vi "PrintTextRead.vi"(0 "No":string, 4 "Time":string, 6 "Date":string, 7 "file path (use dialog)":path=path "E:/NI Program/Merlin try.txt", 8 "Shift":string, 9 "ID":string, 10 "PartNumber":string, 11 "Description":string) -> (1 "FileFound?":bool, 3 "result string":string)   [LabVIEW 2017]
panel:
  in  "PrintMatter":string="\u0010CT~~CD,~CC^~CT~\n^XA~TA080~JSB^LT12^MNW^MTT^PON^PMN^LH0,0^JMA^PR2,2~SD20^JUS^LRN^CI0^XZ\n~DG000.GRF,06400,040,\n,:::::::0FiSFC,0C0iR04,:::::::::::::::::::::::::::::::::::::::::::::::::::::::::::::::::::::::::::::::::::::::::::::::::::::::::::::::::::::::::::::::::::::0FiSFC,:,::::::::::::::^XA\n^MMT\n^PW320\n^LL0152\n^LS0\n^FT0,160^XG000.GRF,1,1^FS\n^FT10,135^A0N,17,16^FH\\^FDDate & Time:^FS\n^FT207,100^A0N,17,16^FH\\^FDID:^FS\n^FT10,98^A0N,17,16^FH\\^FDPart No:^FS\n^FT102,135^A0N,17,16^FH\\^FD01.01.2019 0000^FS\n^FT230,101^A0N,20,19^FH\\^FDoperator^FS\n^FT72,100^A0N,20,19^FH\\^FD123456789^FS\n^FT15,67^A0N,20,19^FH\\^FDFRONT ELECTRIC WR - W501 RH^FS\n^FO4,42^GB297,0,2^FS\n^FT15,31^A0N,17,16^FH\\^FDAditya Auto Products & Engg. (I) Pvt. Ltd.^FS\n^PQ1,0,1,Y^XZ\n^XA^ID000.GRF^FS^XZ\n"
  out "InputText":string
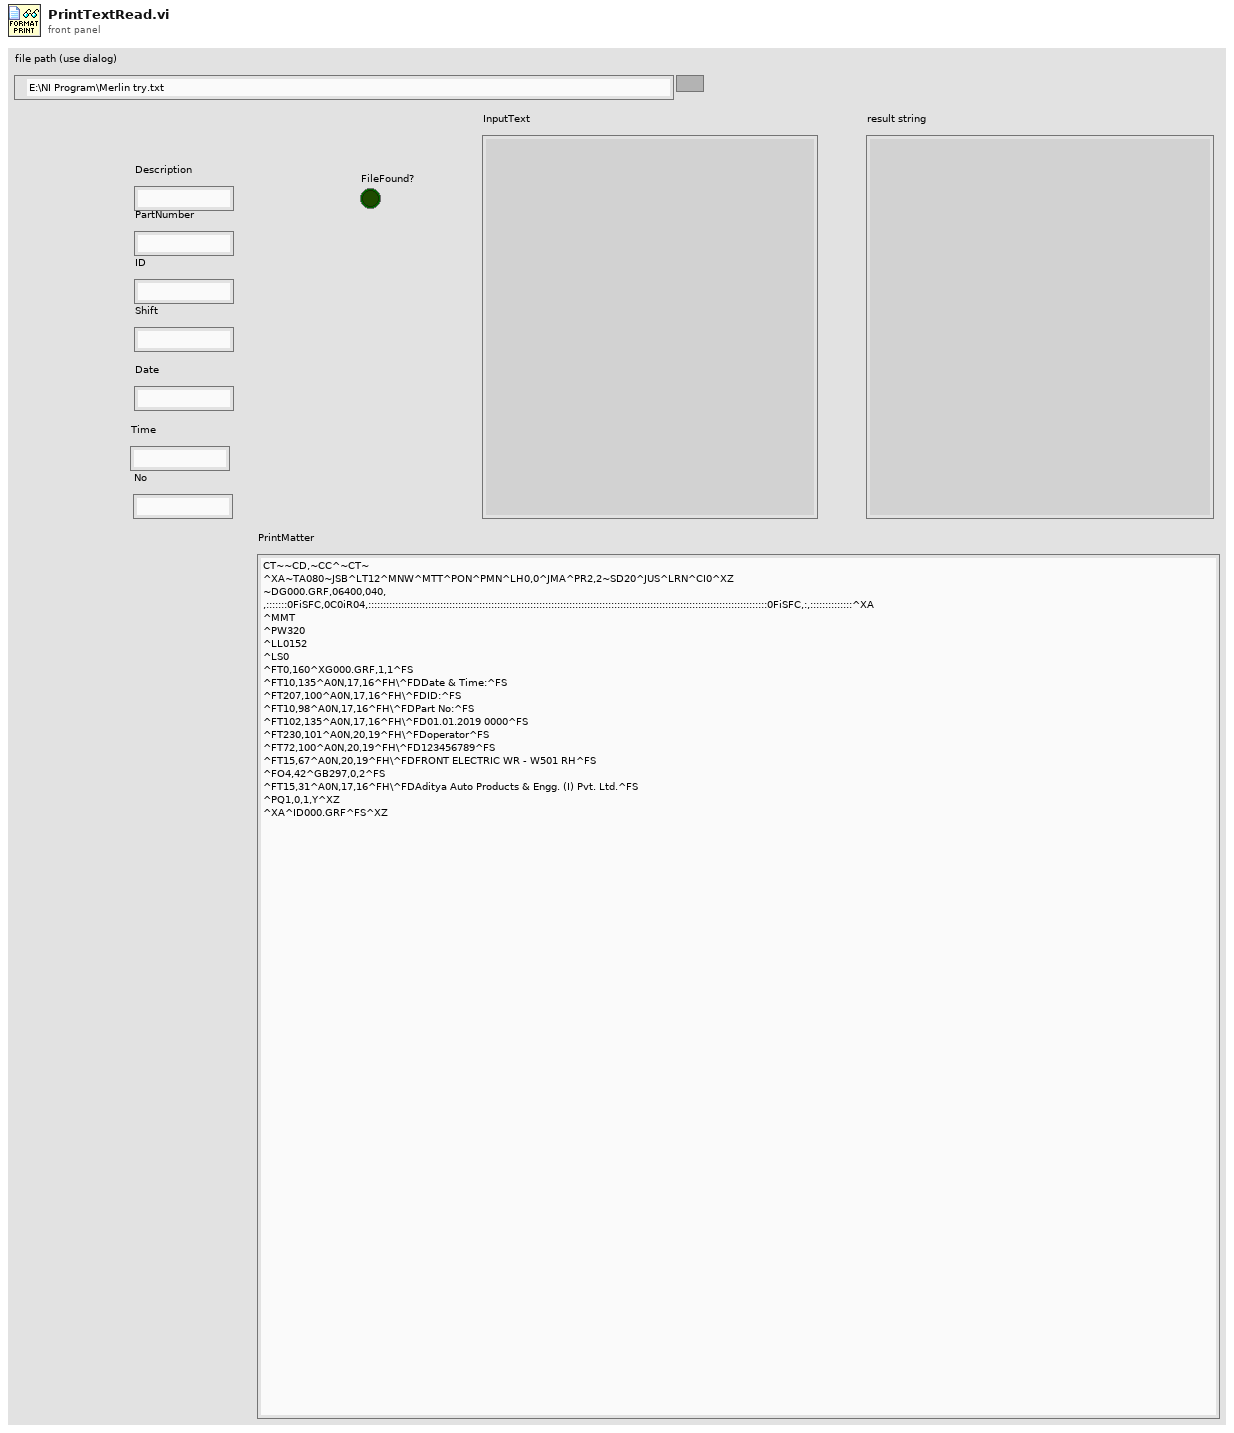
[diagram p1: front panel]
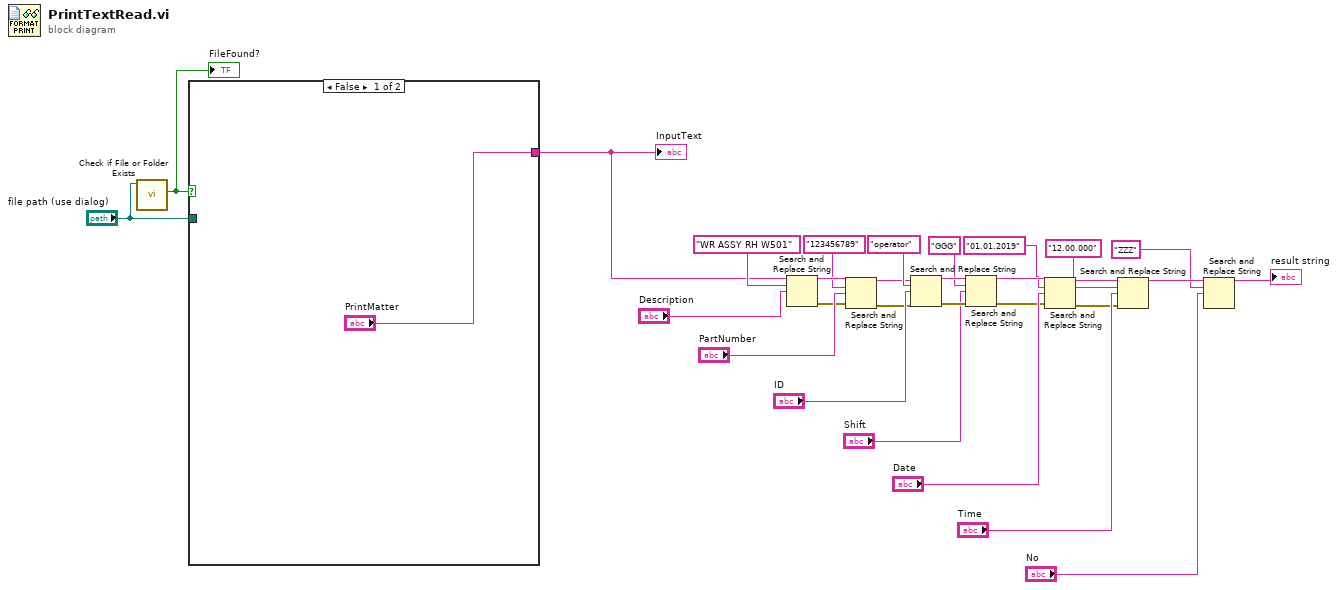
[diagram p0: block diagram]
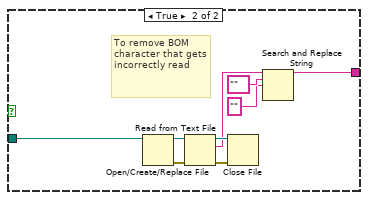
[diagram p2: hidden frame]
diagram:
  n1 = call <vilib>:"Check if File or Folder Exists.vi"("path"="file path (use dialog)") -> ("file or folder exists?"=w15:bool)  [unwired: 8 in, 2 out]
  "FileFound?" <- w15
  n2 = case shown="False" w15 {
    tunnel: ["PrintMatter" w32] -> w21
    tunnel: "file path (use dialog)" -> [_ w31]
    frame False {
    }
    frame True {
      # "To remove BOM character that gets incorrectly read"
      n3 = Open/Create/Replace File(file path (use dialog)=w31) -> (refnum out=w38:refnum<file>, error out=w39:errorcluster)  [unwired: 5 in, 1 out]
      n4 = Read from Text File(file (use dialog)=w38, error in=w39) -> (refnum out=w37:refnum<file>, text=w35:string, error out=w36:errorcluster)  [unwired: 2 in, 1 out]
      n5 = Close File(refnum=w37, error in=w36) -> ()  [unwired: 2 out]
      n6 = Search and Replace String(input string=w35, search string="﻿", replace string="" ("replace string (\"\")")) -> (result string=w32:string)  [unwired: 5 in, 3 out]
    }
  }
  "InputText" <- w21
  n7 = Search and Replace String(input string=w21, search string="WR ASSY RH W501", replace string="Description") -> (result string=w27:string, error out=w24:errorcluster)  [unwired: 5 in, 2 out]
  n8 = Search and Replace String(input string=w27, search string="123456789", replace string="PartNumber", error in=w24) -> (result string=w14:string, error out=w13:errorcluster)  [unwired: 4 in, 2 out]
  n9 = Search and Replace String(input string=w14, search string="operator", replace string="ID", error in=w13) -> (result string=w20:string, error out=w19:errorcluster)  [unwired: 4 in, 2 out]
  n10 = Search and Replace String(input string=w20, search string="GGG", replace string="Shift", error in=w19) -> (result string=w12:string, error out=w7:errorcluster)  [unwired: 4 in, 2 out]
  n11 = Search and Replace String(input string=w12, search string="01.01.2019", replace string="Date", error in=w7) -> (result string=w10:string, error out=w6:errorcluster)  [unwired: 4 in, 2 out]
  n12 = Search and Replace String(input string=w10, search string="12.00.000", replace string="Time", error in=w6) -> (result string=w4:string)  [unwired: 4 in, 3 out]
  n13 = Search and Replace String(input string=w4, search string="ZZZ", replace string="No") -> (result string=→"result string":string)  [unwired: 5 in, 3 out]
